vi "Duration.vi"(8 "error in (no error)":errorcluster, 10 "Duration":dbl, 11 "ModuleID":i32) -> (0 "error out":errorcluster)   [LabVIEW 2018, in "AnalysisModule.lvlib"]
uses:
  AnalysisModule.lvlib
  clEventType.ctl
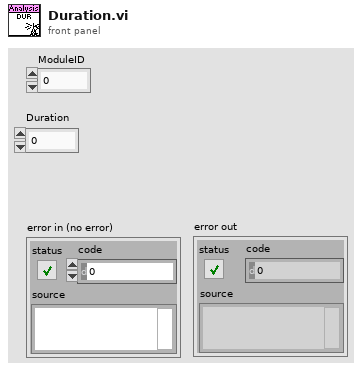
[diagram p1: front panel]
types:
  T1 = typedef "AnalysisModule.lvlib/clEventType.ctl" = cluster{"ModuleID":i32, "Data":variant}
  T2 = typedef "AnalysisModule.lvlib/clBroadcastEvents.ctl" = cluster{"DidInit":refnum<user-event>, "StatusUpdate":refnum<user-event>, "ErrorReport":refnum<user-event>, "DidStop":refnum<user-event>, "PathToINI":refnum<user-event>, "Config":refnum<user-event>, "ResultReport":refnum<user-event>, "FunctionClass":refnum<user-event>, "State":refnum<user-event>, "FunctionParams":refnum<user-event>, "Duration":refnum<user-event>}
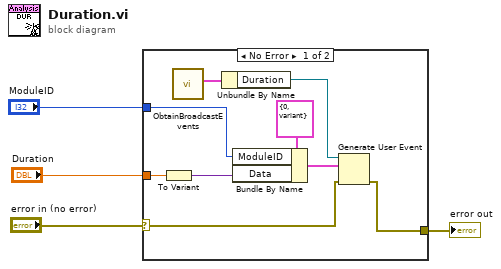
[diagram p0: block diagram]
diagram:
  n1 = case shown="No Error" "error in (no error)" {
    selector: "error in (no error)" -> [w7 w14]
    tunnel: "ModuleID" -> [w12 _]
    tunnel: [w6 w14] -> w3
    tunnel: "Duration" -> [w8 _]
    frame No Error {
      n2 = To Variant(anything=w8) -> (Variant=w5:variant)
      n3 = call "ObtainBroadcastEvents.vi"() -> ("clBroadcastEvents"=w11:T2)  [unwired: 10 in, 1 out]
      n4 = Unbundle By Name(w11) -> ("Duration"=w9:refnum<user-event>)
      n5 = Bundle By Name(cluster=T1 {"ModuleID"=0, "Data"=variant} ("clEventType"), "ModuleID"=w12, "Data"=w5) -> (w10:T1)
      n6 = Generate User Event(user event=w9, event data cluster=w10, error in=w7) -> (error out=w6:errorcluster)  [unwired: 1 in, 1 out]
    }
    frame Error {
    }
  }
  "error out" <- w3
